vi "detekcjazera_final.vi"() -> ()   [LabVIEW 2012]
uses:
  <vilib>/Analysis/3filter.llb/FIR Filter (DBL).vi
  <vilib>/Analysis/baseanly.llb/Mean (DBL).vi
  <vilib>/Utility/file.llb/Read From Spreadsheet File (DBL).vi
  <vilib>/Utility/file.llb/Write To Spreadsheet File (DBL).vi
  <vilib>/Analysis/4window.llb/Hamming Window (DBL).vi
  <vilib>/Analysis/NI_AALBase.lvlib
  <vilib>/Analysis/NI_AALPro.lvlib
  <vilib>/Analysis/NI_AAL_SigProc.lvlib
  <vilib>/gmath/NI_Gmath.lvlib
panel:
  out "Rozpoznano":bool
  out "Zera":dbl[](array[numeric])
  out "Min. indeks":i32
  out "Min. odległość":dbl
  out "Współczynniki":dbl[](array[numeric])
  out "Odległość":dbl[](array[numeric])
  out "Waveform Graph 3":dbl[](graph)
  in  "Liczenie":bool
  in  "Pomiar":bool
  in  "stop":bool
  out "Energia sygnału":dbl
  out "Ramki":dbl[][](array[numeric])
  out "Przekroczenie progu":bool
  out "Tablica ramek":dbl[](graph)
  out "Liczba kolumn":i32
  out "Liczaba wierszy":i32
  out "Energia progowa":dbl
  out "Diagram energii":dbl[](graph)
  out "Wymiar":i32
  out "Suma":dbl
  out "Długość":dbl
  out "Wygładzona energia":dbl[](graph)
  out "Ind. końcowy":dbl
  out "Ind. początkowy":dbl
  out "Wypowiedź":dbl[](graph)
  out "Mowa":waveform(dbl)[](graph)
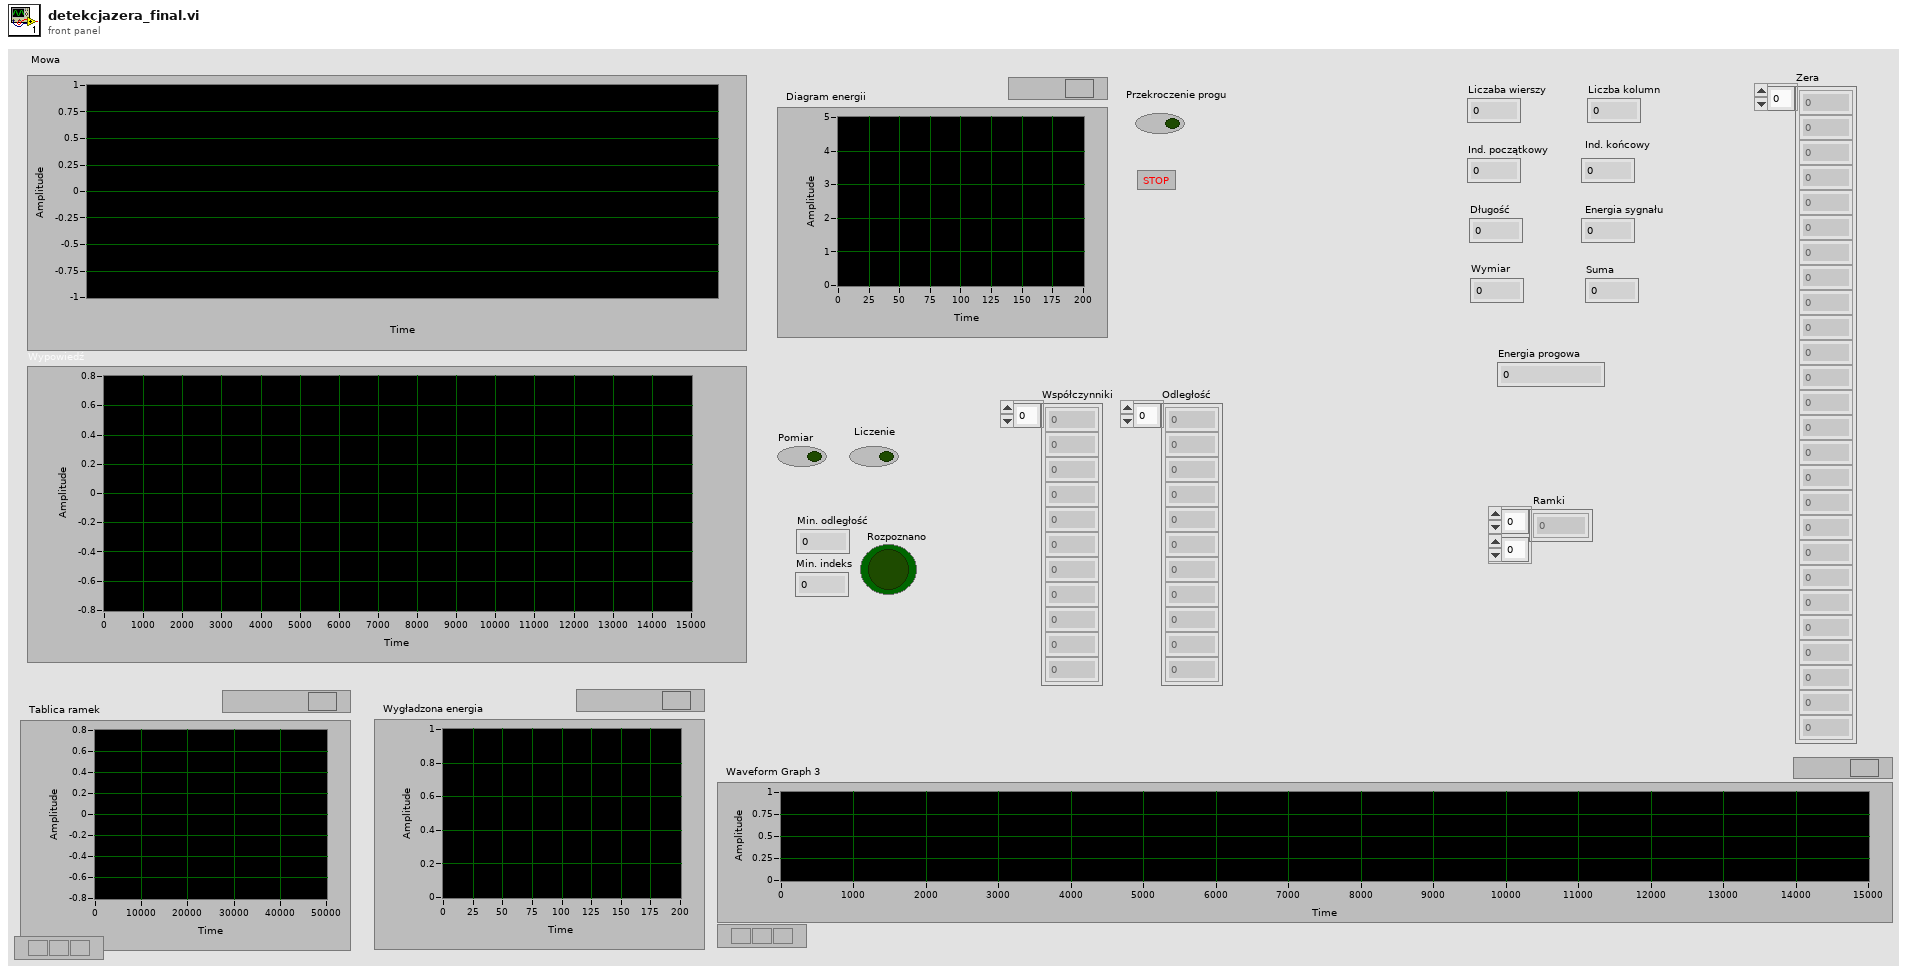
[diagram p1: front panel]
types:
  T1 = enum16{"open", "replace", "create", "open or create", "replace or create", "replace or create with confirmation"}
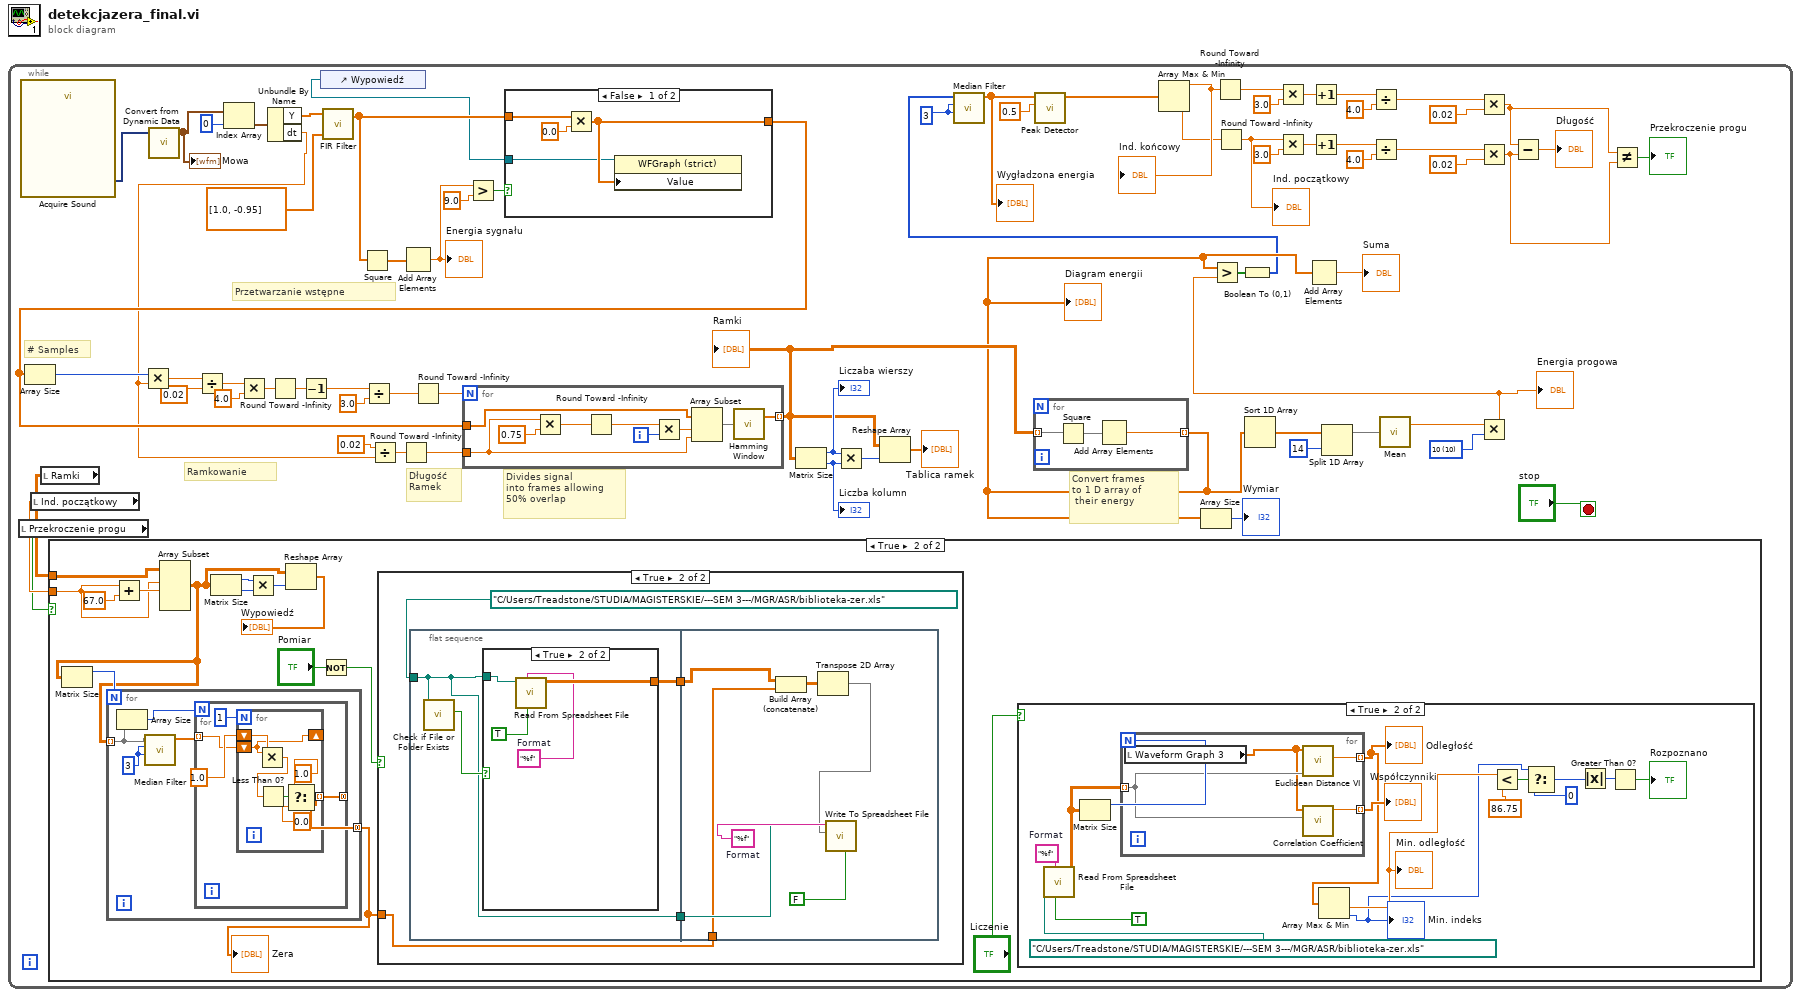
[diagram p0: block diagram]
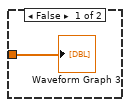
[diagram p3: hidden frame]
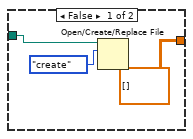
[diagram p4: hidden frame]
diagram:
  n1 = while {
    stop <- "stop" stop-if-true
    w16 = 3 ("right rank")
    w40 = u16 10 items=["5"=5, "6"=6, "7"=7, "9"=9, "10"=10]
    # "Ramkowanie"
    # "Przetwarzanie wstępne"
    # "Convert frames \nto 1 D array of\n their energy"
    # "Divides signal \ninto frames allowing \n50% overlap"
    # "Długość \nRamek"
    # "# Samples"
    n2 = local read "Przekroczenie progu"() -> (w2:bool)
    n3 = call "Acquire Sound"() -> ("Data"=w72:dynamicdata)  [unwired: 18 in, 1 out]
    n4 = local read "Ind. początkowy"() -> (w4:dbl)
    n5 = local read "Ramki"() -> (w3:dbl[][])
    n6 = case shown="True" w2 {
      tunnel: w4 -> [_ w81]
      tunnel: w3 -> [_ w82]
      frame False {
      }
      frame True {
        n7 = Add(x=w81, y=67.0 ("x")) -> (x+y=w85:dbl)
        n8 = Array Subset(array=w82, index (row)=w81, length (row)=w85) -> (w73:dbl[][])  [unwired: 2 in]
        n9 = Matrix Size(0:w73) -> (1:w74:i32)  [unwired: 1 out]
        n10 = for {
          N: w74 -> [_]
          tunnel: [w90] -> w77 mode=concatenating
          tunnel: w73 -> [w88] mode=indexing
          w87 = 3 ("left rank")
          n11 = Array Size(array=w88) -> (size(s)=w91:i32)
          n12 = call <vilib>:"Median Filter.vi"("right rank"=w87, "left rank"=w87, "X"=w88) -> ("Filtered X"=w89:dbl[])  [unwired: 7 in, 1 out]
          n13 = for {
            N: w91 -> [_]
            tunnel: [w95] -> w90 mode=concatenating
            tunnel: w89 -> [w92] mode=indexing
            n14 = for {
              N: 1 -> [_]
              tunnel: [w100] -> w95 mode=indexing
              shift-right: [w96] -> _
              shift-left: 1.0 -> [w98]
              shift-left: w92 -> [w96]
              n15 = Multiply(x=w96, y=w98) -> (x*y=w97:dbl)
              n16 = Less Than 0?(x=w97) -> (x < 0?=w99:bool)
              n17 = Select(t=1.0, s=w99, f=0.0) -> (s? t:f=w100:dbl)
            }
          }
        }
        "Zera" <- w77
        n18 = Matrix Size(0:w73) -> (1:w84:i32, 2:w83:i32)
        n19 = Multiply(x=w84, y=w83) -> (x*y=w76:i32)
        n20 = Reshape Array(w73, w76) -> (→"Wypowiedź":dbl[])
        n21 = Not(x="Pomiar") -> (.not. x?=w78:bool)
        n22 = case shown="True" w78 {
          tunnel: w77 -> [w103 w104]
          frame False {
            "Waveform Graph 3" <- w103
          }
          frame True {
            n23 = flat-sequence {
              tunnel: path "C:/Users/Treadstone/STUDIA/MAGISTERSKIE/---SEM 3---/MGR/ASR/biblioteka-zer.xls" ("file path (dialog if empty)") -> [w108]
              tunnel: [w110] -> w107
              tunnel: [w108] -> w106
              tunnel: w107 -> [w118]
              tunnel: w104 -> [w121]
              tunnel: w106 -> [w122]
              frame #0 {
                n24 = call <vilib>:"Check if File or Folder Exists.vi"("path"=w108) -> ("file or folder exists?"=w109:bool)  [unwired: 8 in, 2 out]
                n25 = case shown="True" w109 {
                  tunnel: w108 -> [w113 w117]
                  tunnel: [dbl[][] [] ("all rows") w116] -> w110
                  frame False {
                    n26 = Open/Create/Replace File(file path (use dialog)=w113, operation (0:open)=T1."create") -> ()  [unwired: 4 in, 3 out]
                  }
                  frame True {
                    w115 = "%f"  # Format
                    n27 = call-poly <vilib>:"Read From Spreadsheet File.vi"("transpose (no:F)"=TRUE, "format (%.3f)"=w115, "file path (dialog if empty)"=w117) -> ("all rows"=w116:dbl[][])  [unwired: 4 in, 4 out]
                  }
                }
              }
              frame #1 {
                w124 = "%f"  # Format
                n28 = Build Array (concatenate)(w118, w121) -> (w120:dbl[][])
                n29 = Transpose 2D Array(2D array=w120) -> (transposed array=w119:dbl[][])
                n30 = call-poly <vilib>:"Write To Spreadsheet File.vi"("transpose? (no:F)"=FALSE, "format (%.3f)"=w124, "2D data"=w119, "file path (dialog if empty)"=w122) -> ()  [unwired: 4 in, 1 out]
              }
            }
          }
        }
        n31 = case shown="True" "Liczenie" {
          frame False {
          }
          frame True {
            w138 = "%f"  # Format
            n32 = call-poly <vilib>:"Read From Spreadsheet File.vi"("transpose (no:F)"=TRUE, "format (%.3f)"=w138, "file path (dialog if empty)"=path "C:/Users/Treadstone/STUDIA/MAGISTERSKIE/---SEM 3---/MGR/ASR/biblioteka-zer.xls") -> ("all rows"=w134:dbl[][])  [unwired: 4 in, 4 out]
            n33 = Matrix Size(0:w134) -> (1:w136:i32)  [unwired: 1 out]
            n34 = for {
              N: w136 -> [_]
              tunnel: w134 -> [w143] mode=indexing
              tunnel: [w141] -> w133 mode=indexing
              tunnel: [w140] -> w135 mode=indexing
              n35 = local read "Waveform Graph 3"() -> (w142:dbl[])
              n36 = call "Euclidean Distance VI.vi"("Reference"=w143, "Test"=w142) -> ("Dist"=w141:dbl)  [unwired: 9 in]
              n37 = call <vilib>:"Correlation Coefficient.vi"("Y"=w143, "X"=w142) -> ("correlation coefficient r"=w140:dbl)  [unwired: 8 in, 1 out]
            }
            "Odległość" <- w133
            "Współczynniki" <- w135
            n38 = Array Max & Min(array=w133) -> (min value=w126:dbl, min index (indices)=w125:i32)  [unwired: 2 out]
            "Min. odległość" <- w126
            "Min. indeks" <- w125
            n39 = Less?(x=w126, y=86.75) -> (x < y?=w132:bool)
            n40 = Select(t=w125, s=w132, f=0) -> (s? t:f=w130:i32)
            n41 = Absolute Value(x=w130) -> (abs(x)=w129:i32)
            n42 = Greater Than 0?(x=w129) -> (x > 0?=→"Rozpoznano":bool)
          }
        }
      }
    }
    n43 = call "Convert from Dynamic Data"("Dynamic Data Type"=w72) -> ("Array of Waveform"=w1:waveform(dbl)[])  [unwired: 3 in]
    "Mowa" <- w1
    n44 = Index Array(array=w1, index=0) -> (element=w62:waveform(dbl))
    n45 = Unbundle By Name(w62) -> ("Y"=w61:dbl[], "dt"=w41:dbl)
    n46 = control-ref of="Wypowiedź"() -> (w5:refnum<vi>)
    n47 = call-poly <vilib>:"FIR Filter.vi"("FIR Coefficients"=dbl[] [1.0, -0.95], "X"=w61) -> ("Filtered X"=w70:dbl[])  [unwired: 2 in, 1 out]
    n48 = Square(x=w70) -> (x^2=w66:dbl[])
    n49 = Divide(x=0.02, y=w41) -> (x/y=w47:dbl)
    n50 = Round Toward -Infinity(1:w47) -> (0:w48:dbl)
    n51 = Add Array Elements(numeric array=w66) -> (sum=w68:dbl)
    "Energia sygnału" <- w68
    n52 = Greater?(x=w68, y=9.0) -> (0:w69:bool)
    n53 = case shown="False" w69 {
      tunnel: w70 -> [w158 w160]
      tunnel: [w157 w160] -> w42
      tunnel: w5 -> [w156 _]
      frame False {
        n54 = Multiply(x=w158, y=0.0) -> (x*y=w157:dbl[])
        n55 = property class="WFGraph (strict)"(reference=w156, "Value"=w157) -> ()  [unwired: 1 in, 2 out]
      }
      frame True {
      }
    }
    n56 = Array Size(array=w42) -> (size(s)=w60:i32)
    n57 = Multiply(x=w60, y=w41) -> (x*y=w58:dbl)
    n58 = Divide(x=w58, y=0.02) -> (x/y=w54:dbl)
    n59 = Multiply(x=w54, y=4.0) -> (x*y=w53:dbl)
    n60 = Round Toward -Infinity(1:w53) -> (0:w56:dbl)
    n61 = Decrement(x=w56) -> (x-1=w51:dbl)
    n62 = Divide(x=w51, y=3.0) -> (x/y=w50:dbl)
    n63 = Round Toward -Infinity(1:w50) -> (0:w49:dbl)
    n64 = for {
      N: w49 -> [_]
      tunnel: w42 -> [w155]
      tunnel: w48 -> [w152]
      tunnel: [w147] -> w32 mode=indexing
      i -> [w154]
      n65 = Multiply(x=w152, y=0.75 ("x")) -> (x*y=w150:dbl)
      n66 = Round Toward -Infinity(1:w150) -> (0:w149:dbl)
      n67 = Multiply(x=w149, y=w154) -> (x*y=w151:dbl)
      n68 = Array Subset(array=w155, index=w151, length=w152) -> (w148:dbl[])
      n69 = call-poly <vilib>:"Hamming Window.vi"("X"=w148) -> ("Windowed X"=w147:dbl[])  [unwired: 1 out]
    }
    "Ramki" <- w32
    n70 = Matrix Size(0:w32) -> (1:w46:i32, 2:w45:i32)
    "Liczba kolumn" <- w45
    "Liczaba wierszy" <- w46
    n71 = Multiply(x=w46, y=w45) -> (x*y=w44:i32)
    n72 = Reshape Array(w32, w44) -> (→"Tablica ramek":dbl[])
    n73 = for {
      tunnel: w32 -> [w146] mode=indexing
      tunnel: [w144] -> w9 mode=indexing
      n74 = Square(x=w146) -> (x^2=w145:dbl[])
      n75 = Add Array Elements(numeric array=w145) -> (sum=w144:dbl)
    }
    "Diagram energii" <- w9
    n76 = Array Size(array=w9) -> (size(s)=→"Wymiar":i32)
    n77 = Sort 1D Array(array=w9) -> (sorted array=w36:dbl[])
    n78 = Add Array Elements(numeric array=w9) -> (sum=→"Suma":dbl)
    n79 = Split 1D Array(array=w36, index=14) -> (first subarray=w34:dbl[])  [unwired: 1 out]
    n80 = call-poly <vilib>:"Mean.vi"("X"=w34) -> ("mean"=w33:dbl)  [unwired: 1 out]
    n81 = Multiply(x=w33, y=w40) -> (x*y=w39:dbl)
    "Energia progowa" <- w39
    n82 = Greater?(x=w9, y=w39) -> (0:w38:bool[])
    n83 = Boolean To (0,1)(Boolean=w38) -> (0, 1=w6:i16[])
    n84 = call <vilib>:"Median Filter.vi"("right rank"=w16, "left rank"=w16, "X"=w6) -> ("Filtered X"=w13:dbl[])  [unwired: 7 in, 1 out]
    "Wygładzona energia" <- w13
    n85 = call <vilib>:"Peak Detector.vi"("threshold"=0.5, "X"=w13) -> ("Locations"=w15:dbl[])  [unwired: 5 in, 4 out]
    n86 = Array Max & Min(array=w15) -> (max value=w17:dbl, min value=w12:dbl)  [unwired: 2 out]
    "Ind. końcowy" <- w17
    n87 = Round Toward -Infinity(1:w17) -> (0:w30:dbl)
    n88 = Round Toward -Infinity(1:w12) -> (0:w11:dbl)
    "Ind. początkowy" <- w11
    n89 = Multiply(x=w30, y=3.0) -> (x*y=w19:dbl)
    n90 = Multiply(x=w11, y=3.0) -> (x*y=w28:dbl)
    n91 = Increment(x=w19) -> (x+1=w20:dbl)
    n92 = Increment(x=w28) -> (x+1=w27:dbl)
    n93 = Divide(x=w20, y=4.0) -> (x/y=w22:dbl)
    n94 = Divide(x=w27, y=4.0) -> (x/y=w25:dbl)
    n95 = Multiply(x=w22, y=0.02) -> (x*y=w8:dbl)
    n96 = Multiply(x=w25, y=0.02) -> (x*y=w7:dbl)
    n97 = Subtract(x=w8, y=w7) -> (x-y=→"Długość":dbl)
    n98 = Not Equal?(x=w8, y=w7) -> (x != y?=→"Przekroczenie progu":bool)
  }
